vi "SetEntryRepetitions.vi"(1 "Entry Repetitions Options":u16(ring) items=["Value", "Default", "Minimum", "Maximum", "Infinite"], 3 "error in (no error)":errorcluster, 4 "Entry Repetitions (N)":i32=1 min=1, 5 "Element":i16=1 min=1, 6 "VISA resource name":refnum<visa-resource-name>) -> (0 "error out":errorcluster, 2 "VISA resource name out":refnum<visa-resource-name>)   [LabVIEW 2020, in "Active Technologies AWG3000.lvlib"]
uses:
  Active Technologies AWG3000.lvlib
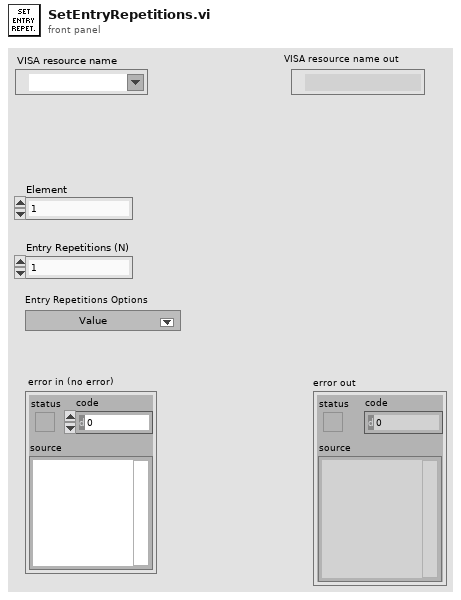
[diagram p1: front panel]
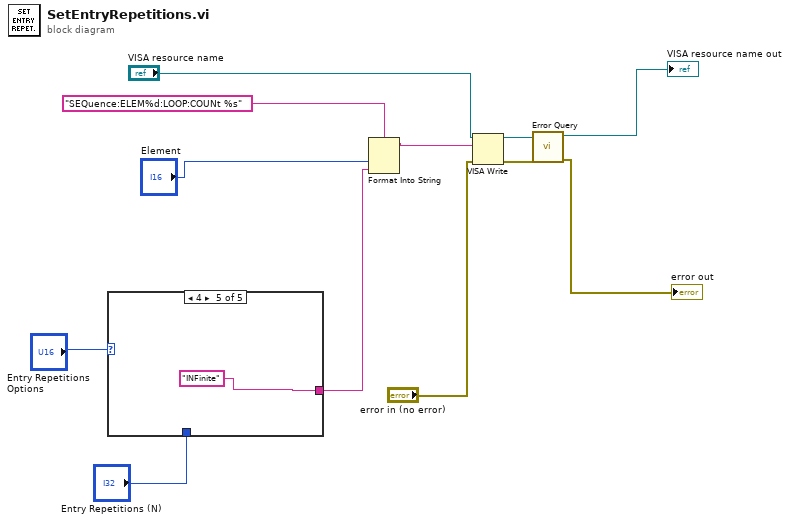
[diagram p0: block diagram]
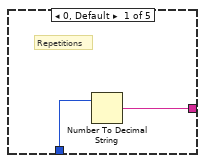
[diagram p2: hidden frame]
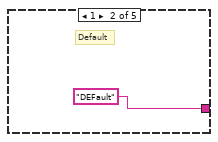
[diagram p3: hidden frame]
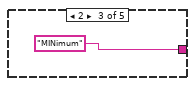
[diagram p4: hidden frame]
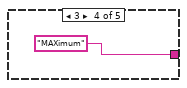
[diagram p5: hidden frame]
diagram:
  n1 = case shown="4" "Entry Repetitions Options" {
    tunnel: [w14 "DEFault" ("write buffer") "MINimum" ("write buffer") "MAXimum" ("write buffer") "INFinite" ("write buffer")] -> w1
    tunnel: "Entry Repetitions (N)" -> [w13 _ _ _ _]
    frame 0, Default {
      # "Repetitions"
      n2 = Number To Decimal String(number=w13) -> (decimal integer string=w14:string)  [unwired: 1 in]
    }
    frame 1 {
      # "Default"
    }
    frame 2 {
    }
    frame 3 {
    }
    frame 4 {
    }
  }
  n3 = Format Into String(format string="SEQuence:ELEM%d:LOOP:COUNt %s" ("write buffer"), "Element", w1) -> (resulting string=w2:string)  [unwired: 2 in, 1 out]
  n4 = VISA Write(VISA resource name="VISA resource name", write buffer=w2, error in (no error)="error in (no error)") -> (VISA resource name out=w9:refnum<visa-resource-name>, error out=w8:errorcluster)  [unwired: 1 out]
  n5 = call "Error Query.vi"("error in (no error)"=w8, "VISA resource name"=w9) -> ("error out"=→"error out":errorcluster, "VISA resource name out"=→"VISA resource name out":refnum<visa-resource-name>)  [unwired: 6 in, 2 out]
